vi "Top-Level-Test.vi"() -> ()   [LabVIEW 2016]
uses:
  <vilib>/rvi/interface/RandomDataEmulation/nirviRandomDataOpen.vi
  <vilib>/rvi/interface/common/niFpgaCacheSessionInfoDynamic.vi
  <vilib>/Utility/error.llb/Error Cluster From Error Code.vi
  <vilib>/rvi/errors/niLvFpgaAdjustHostInterfaceError.vi
  <vilib>/FPGAPlugInAG/Dynamic/niLvFpga_Close_Dynamic.vi
  <vilib>/rvi/interface/nirviOpenFPGA/nirviOpenFPGA.xnode
  Fpga/Fpga-Test-Harness.vi
  <vilib>/rvi/interface/nirviReadWriteControl/nirviReadWriteControl.xnode
  <vilib>/rvi/interface/nirviMethod/nirviMethod.xnode
  <vilib>/rvi/interface/nirviCloseFPGA/nirviCloseFPGA.xnode
  <vilib>/FPGAPlugInAG/Dynamic/niLvFpga_WriteFifo_Dynamic.vi
  <vilib>/rvi/errors/niLvFpgaMergeErrorWithErrorCode.vi
  <vilib>/FPGAPlugInAG/Dynamic/niLvFpga_ReadFifo_Dynamic.vi
  NiFpgaLv.dll
  <vilib>/rvi/interface/Simulation/niFpgaSimulationCallBeginRW.vi
panel:
  in  "Operating\nMode":enum16{"OrderBook"}(ring)
  out "DataOut":u64[](array[numeric]) format="%.0x"
  out "error out":errorcluster
  in  "DataIn":u64[](array[numeric]) format="%.0x"
  in  "error in":errorcluster
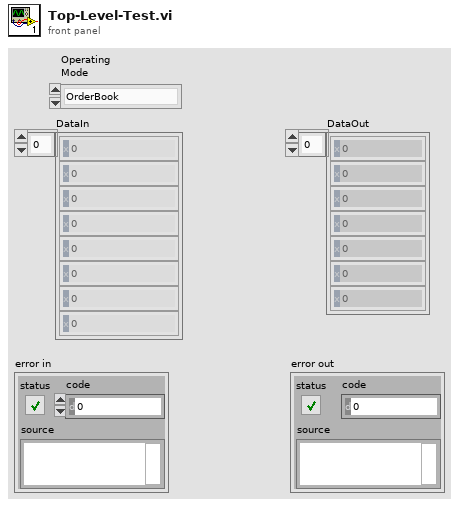
[diagram p1: front panel]
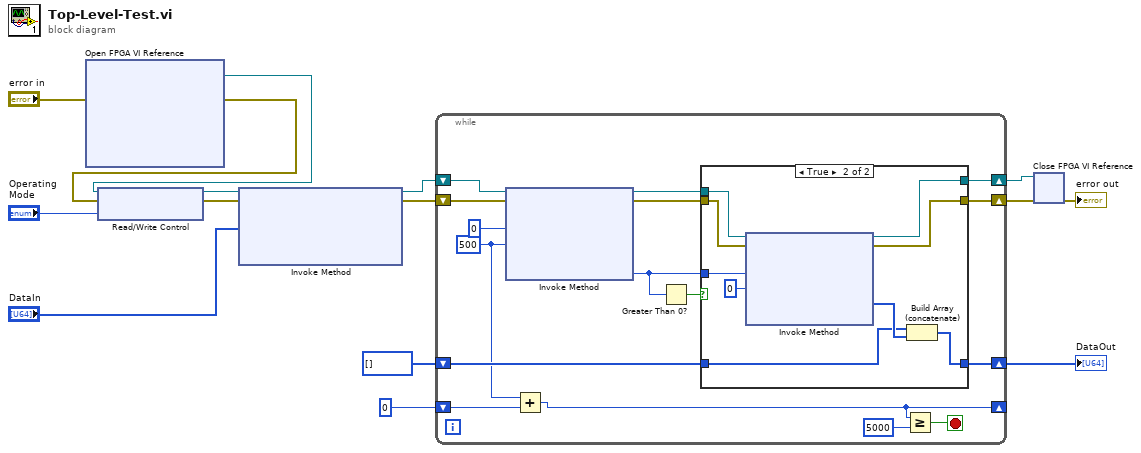
[diagram p0: block diagram]
diagram:
  n1 = xnode "Open FPGA VI Reference"("error in"="error in") -> ("FPGA VI Reference Out"=w14:refnum<k20>, "error out"=w5:errorcluster)  [unwired: 1 in]
  n2 = xnode "Read/Write Control"("FPGA VI Reference In"=w14, "error in"=w5, "Operating Mode"="Operating\nMode") -> ("FPGA VI Reference Out"=w6:refnum<k20>, "error out"=w4:errorcluster)
  n3 = xnode "Invoke Method"("FPGA VI Reference In"=w6, "error in"=w4, "Data"="DataIn") -> ("FPGA VI Reference Out"=w12:refnum<k20>, "error out"=w11:errorcluster)  [unwired: 1 in, 1 out]
  n4 = while {
    shift-right: [w24] -> w1
    shift-left: w12 -> [w31]
    shift-right: [w23] -> w9
    shift-left: w11 -> [w30]
    shift-right: [w16] -> w2
    shift-left: u64[] [] -> [w22]
    shift-right: [w19] -> _
    shift-left: 0 ("Timeout (ms)") -> [w20]
    stop <- w17 stop-if-true
    w21 = 500 ("Timeout (ms)")
    n5 = xnode "Invoke Method"("FPGA VI Reference In"=w31, "error in"=w30, "Number of Elements"=u32 0, "Timeout (ms)"=w21) -> ("FPGA VI Reference Out"=w25:refnum<k20>, "error out"=w26:errorcluster, "Elements Remaining"=w27:u32)  [unwired: 1 out]
    n6 = Add(x=w21, y=w20) -> (x+y=w19:i32)
    n7 = Greater Than 0?(x=w27) -> (x > 0?=w28:bool)
    n8 = case shown="True" w28 {
      tunnel: w27 -> [_ w43]
      tunnel: w26 -> [w33 w42]
      tunnel: w25 -> [w34 w41]
      tunnel: [w34 w40] -> w24
      tunnel: [w33 w39] -> w23
      tunnel: w22 -> [w32 w36]
      tunnel: [w32 w35] -> w16
      frame False {
      }
      frame True {
        n9 = xnode "Invoke Method"("FPGA VI Reference In"=w41, "error in"=w42, "Number of Elements"=w43, "Timeout (ms)"=0) -> ("FPGA VI Reference Out"=w40:refnum<k20>, "error out"=w39:errorcluster, "Data"=w37:u64[])  [unwired: 1 out]
        n10 = Build Array (concatenate)(w36, w37) -> (w35:u64[])
      }
    }
    n11 = Greater Or Equal?(x=w19, y=5000) -> (x >= y?=w17:bool)
  }
  "DataOut" <- w2
  n12 = xnode "Close FPGA VI Reference"("FPGA VI Reference In"=w1, "error in"=w9) -> ("error out"=→"error out":errorcluster)
